vi "Laser-Scan.vi"(7 "Scan":bool, 8 "Step":dbl=0.01 format="%#_13g", 9 "Final":dbl=227.0 format="%#_13g", 10 "Initial":dbl=226.0 format="%#_13g", 11 "COM4":refnum<visa-resource-name>="COM4") -> (2 "Current Lambda (cm-1)":dbl, 3 "Current Lambda (nm)":dbl format="%.2f")   [LabVIEW 2018]
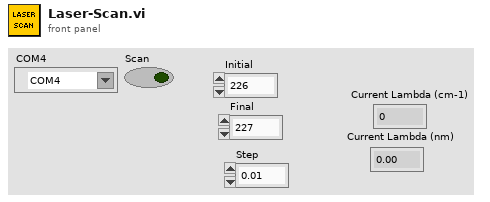
[diagram p1: front panel]
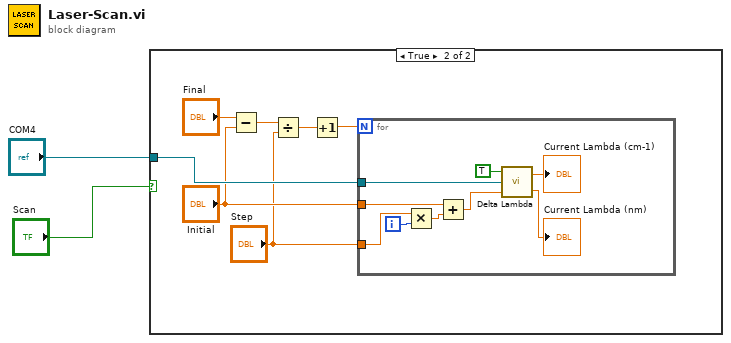
[diagram p0: block diagram]
diagram:
  n1 = case shown="True" "Scan" {
    tunnel: "COM4" -> [_ w9]
    frame False {
    }
    frame True {
      n2 = Subtract(x="Final", y="Initial") -> (x-y=w6:dbl)
      n3 = Divide(x=w6, y="Step") -> (x/y=w4:dbl)
      n4 = Increment(x=w4) -> (x+1=w3:dbl)
      n5 = for {
        N: w3 -> [_]
        tunnel: w9 -> [w18]
        tunnel: "Step" -> [w17]
        tunnel: "Initial" -> [w14]
        i -> [w15]
        n6 = Multiply(x=w17, y=w15) -> (x*y=w16:dbl)
        n7 = Add(x=w14, y=w16) -> (x+y=w13:dbl)
        n8 = call "Delta Lambda.vi"("Change Lambda (nm) to:"=w13, "COM4"=w18, "Boolean"=TRUE) -> ("New Lambda (nm)"=→"Current Lambda (nm)":dbl, "New Lambda (cm-1)"=→"Current Lambda (cm-1)":dbl)
      }
    }
  }
